vi "adjust.vi"(8 "error in (no error)":errorcluster, 11 "GenericLightSource in":refnum<class "GenericLightSource.lvclass">) -> (0 "error out":errorcluster, 3 "GenericLightSource out":refnum<class "GenericLightSource.lvclass">)   [LabVIEW 2010, in "GenericLightSource.lvclass"]
uses:
  GenericLightSource.lvclass
panel:
  # "This functionality is not implemented for this component."
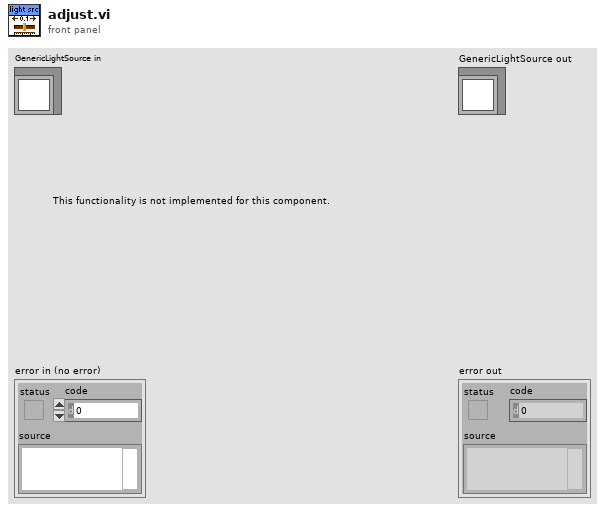
[diagram p1: front panel]
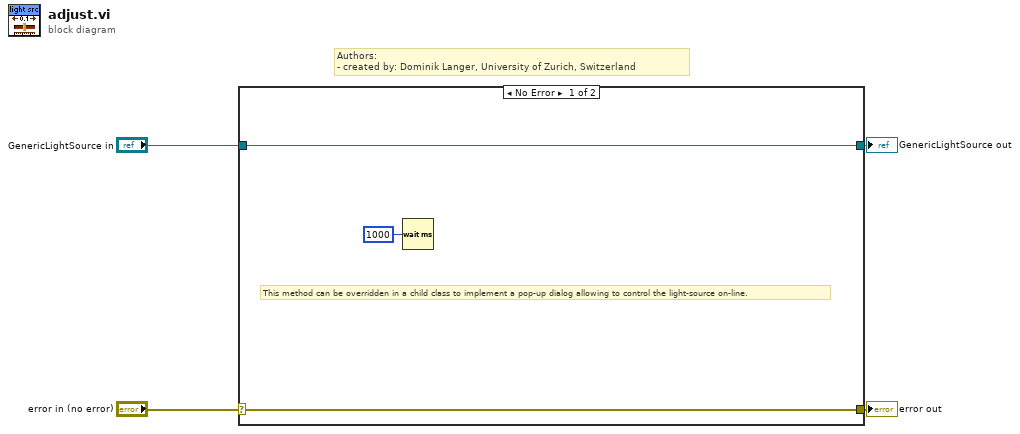
[diagram p0: block diagram]
diagram:
  # "Authors: \n- created by: Dominik Langer, University of Zurich, Switzerland"
  n1 = case shown="No Error" "error in (no error)" {
    selector: "error in (no error)" -> [w6 w9]
    tunnel: [w6 w9] -> w3
    tunnel: [w7 w8] -> w1
    tunnel: "GenericLightSource in" -> [w7 w8]
    frame No Error {
      # "This method can be overridden in a child class to implement a pop-up dialog allowing to control the light-source on-line."
      n2 = Wait (ms)(milliseconds to wait=u32 1000) -> ()  [unwired: 1 out]
    }
    frame Error {
    }
  }
  "error out" <- w3
  "GenericLightSource out" <- w1
